vi "Validate Channel or Array Name.vi"(8 "Error In":errorcluster, 10 "Name in":string, 11 "Message Refnum In":T1 format="%.0x") -> (0 "Error Out":errorcluster, 2 "Name Out":string, 3 "Message Refnum Out":T1 format="%.0x")   [LabVIEW 2018, in "Instrument Addon Scripting API.lvlib"]
doc: "Verifies if the desired channel/array name is already in use.\n\nInput: \nMessage Refnum In: represents the reference to the \"Response\" message section.\nName In: represents the desired name for the Data Channel/Data Array.\n\nOutput:\nMessage Refnum Out: represents the reference to the \"Response\" message section provided as input.\nName Out: represents the desired name provided as input."
uses:
  Instrument Addon Scripting API.lvlib
  <vilib>/NI Veristand/Custom Device API/Custom Device Item Ref.ctl
  NationalInstruments.VeriStand.SystemDefinitionAPI
  Addon/Addon Shared/SubVIs/Constants.vi
  <vilib>/NI/NI VeriStand Advanced SysDef API/_SubVIs/SysDef.Search.GUIDs.vi
  <vilib>/Utility/error.llb/Error Cluster From Error Code.vi
  <vilib>/ErrorRing/Error Ring.xnode
  <vilib>/NI/NI VeriStand Advanced SysDef API/SysDef API/Advanced System Definition.lvlib
  Addon/Addon Shared/Instrument Addon Shared.lvlib
  <vilib>/NI Veristand/Custom Device API/Custom Device API.lvlib
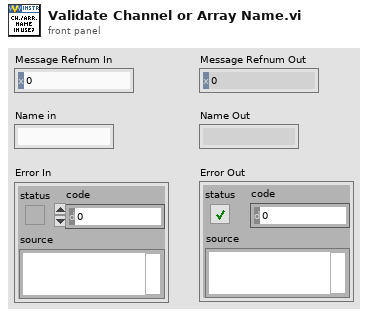
[diagram p1: front panel]
types:
  T1 = typedef "Custom Device API.lvlib/Custom Device Item Ref.ctl" = u64
  T2 = typedef "Advanced System Definition.lvlib/TreeItem.Info.ctl" = cluster{"Name":string, "Description":string, "GUID":string, "Is Channel":bool, "Channel":T3, "Is Waveform":bool, "Waveform":T5}
  T3 = typedef "Custom Device API.lvlib/Custom Device Channel.ctl" = cluster{"Type":T4, "Units":string, "Default Value":dbl, "Faultable":bool, "Scalable":bool}
  T4 = typedef "Custom Device API.lvlib/Custom Device Channel Type.ctl" = enum16{"Input", "Output"}
  T5 = typedef "Custom Device API.lvlib/Custom Device Waveform.ctl" = cluster{"Data Type":T6, "Units":string}
  T6 = typedef "Custom Device API.lvlib/Custom Device Waveform DataType.ctl" = enum16{"Double", "Complex Double"}
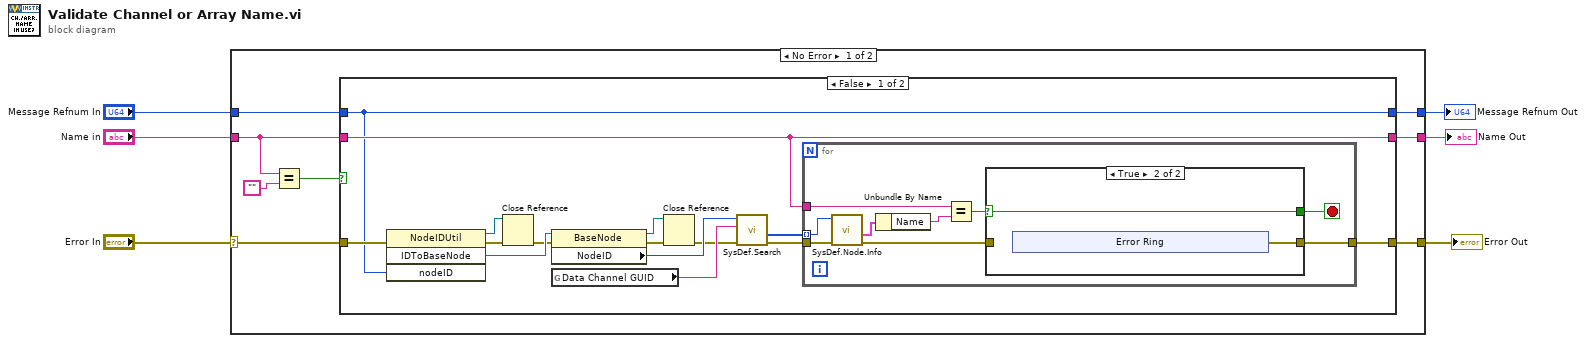
[diagram p0: block diagram]
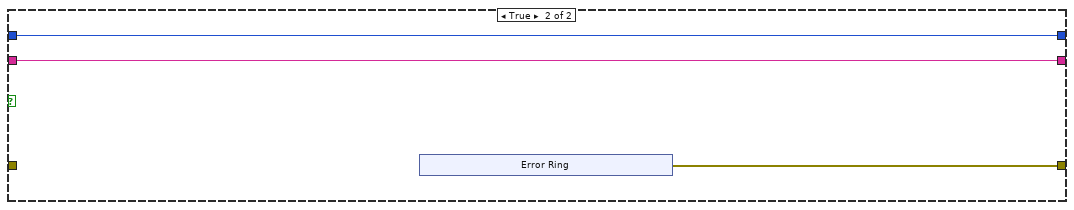
[diagram p3: hidden frame]
diagram:
  n1 = case shown="No Error" "Error In" {
    selector: "Error In" -> [w13 w57]
    tunnel: "Name in" -> [w8 w56]
    tunnel: "Message Refnum In" -> [w12 w58]
    tunnel: [w11 w58] -> w3
    tunnel: [w9 w57] -> w1
    tunnel: [w7 w56] -> w2
    frame No Error {
      n2 = Equal?(x=w8, y="") -> (x = y?=w10:bool)
      n3 = case shown="False" w10 {
        tunnel: w13 -> [w21 _]
        tunnel: w12 -> [w15 w49]
        tunnel: [w15 w49] -> w11
        tunnel: [w17 w50] -> w9
        tunnel: w8 -> [w16 w48]
        tunnel: [w16 w48] -> w7
        frame False {
          n4 = invoke class="NodeIDUtil" method="IDToBaseNode"(error in=w21, "nodeID"=w15) -> (reference out=w25:refnum<k24>, error out=w27:errorcluster, "IDToBaseNode"=w29:refnum<k24>)  [unwired: 2 in, 1 out]
          n5 = Close Reference(reference=w25, error in (no error)=w27) -> (error out=w26:errorcluster)
          n6 = property class="BaseNode"(reference=w29, error in=w26) -> (reference out=w23:refnum<k24>, error out=w24:errorcluster, "NodeID"=w28:u64)
          n7 = global read "Constants.vi" "Data Channel GUID"() -> (w22:string)
          n8 = Close Reference(reference=w23, error in (no error)=w24) -> (error out=w20:errorcluster)
          n9 = call-poly <vilib>:"SysDef.Search.vi"("error in (no error)"=w20, "GUID"=w22, "nodeID"=w28) -> ("error out"=w19:errorcluster, "Values Out"=w18:u64[])  [unwired: 5 in, 2 out]
          n10 = for {
            tunnel: w19 -> [w38]
            tunnel: w18 -> [w37] mode=indexing
            tunnel: w16 -> [w35]
            tunnel: [w32] -> w17
            stop <- w30 stop-if-true
            n11 = call <vilib>:"SysDef.Node.Info.vi"("error in (no error)"=w38, "nodeID"=w37) -> ("error out"=w31:errorcluster, "Item Info"=w36:T2)  [unwired: 6 in, 2 out]
            n12 = Unbundle By Name(w36) -> ("Name"=w34:string)
            n13 = Equal?(x=w35, y=w34) -> (x = y?=w33:bool)
            n14 = case shown="True" w33 {
              selector: w33 -> [w39 w41]
              tunnel: [w40 w42] -> w32
              tunnel: w31 -> [w40 _]
              tunnel: [w39 w41] -> w30
              frame False {
              }
              frame True {
                n15 = xnode "Error Ring"() -> ("error out"=w42:errorcluster)
              }
            }
          }
        }
        frame True {
          n16 = xnode "Error Ring"() -> ("error out"=w50:errorcluster)
        }
      }
    }
    frame Error {
    }
  }
  "Message Refnum Out" <- w3
  "Name Out" <- w2
  "Error Out" <- w1
